vi "WLC Fitting For OneDirectionOnly_YCC.vi"() -> ()   [LabVIEW 2014]
uses:
  SubVI/WLC-Fitting Cluster.ctl
  <vilib>/Utility/file.llb/Read From Spreadsheet File (DBL).vi
  <vilib>/gmath/NumericalOptimization/Nonlinear Curve Fit LM formula string.vi
  <vilib>/Utility/file.llb/Write To Spreadsheet File (DBL).vi
  <vilib>/gmath/NI_Gmath.lvlib
panel:
  out "F-Force":dbl[](array[numeric])
  out "F-xDNA":dbl[](array[numeric])
  in  "F-yr shift (mV)":dbl
  in  "F-cr shift (nm)":dbl
  out "F-QPD signal (V)":dbl[](array[numeric])
  out "F-Stage Positions (um)":dbl[](array[numeric])
  in  "stuckbead path (dialog if empty)":path
  in  "F+U data?":bool
  in  "Ready to Fit":bool
  out "Save to Path":path
  out "best nonlinear fit force":dbl[](array[numeric])
  in  "SaveName":enum16{"ForecExtension Only", "WLC Fitting"}(ring)
  in  "Save Data?":bool
  in  "Finish Fitting":bool
  out "best fit parameters":dbl[](array[numeric])
  in  "initial parameters 2":dbl[](array[numeric])=[40.0, 1150.0]
  in  "Enum":T1(ring)
  in  "initial parameters for fit K":dbl[](array[numeric])=[40.0, 1150.0]
  out "U-Force":dbl[](array[numeric])
  out "U-xDNA":dbl[](array[numeric])
  out "Fitting Cluster for indicator":T2={"cr (um)"=0.0, "yr (V)"=0.0, "trap height(nm)"=0.0, "bead radius(nm)"=520.0, "Length offset"=0.0, "Force offset"=0.0, "cr shift (nm)"=0.0, "yr shift (mV)"=0.0, "LaserPower (mW)"=0.0, "conversion factor (V/um)"=0.0, "Stiffness (pN/nm)"=0.0154}
  in  "OneDirectionOnly?":bool=TRUE
  in  "Fitting Cluster for contorl":T2={"cr (um)"=0.0, "yr (V)"=0.0, "trap height(nm)"=200.0, "bead radius(nm)"=520.0, "Length offset"=0.0, "Force offset"=0.0, "cr shift (nm)"=0.0, "yr shift (mV)"=0.0, "LaserPower (mW)"=0.0, "conversion factor (V/um)"=0.0, "Stiffness (pN/nm)"=0.0154}
  in  "Tab Control":T3(tab)
  out "Stage-QPD Graph":T4(graph)
  out "U-Extension-Force Graph":cluster{"xDNA":dbl[], "Force":dbl[]}(graph)
  out "F-Extension-Force Graph":cluster{"xDNA":dbl[], "Force":dbl[]}(graph)
  out "All-Extension-Force Graph":T5(graph)
  out "Extension-Force and WLC Graph":cluster{"xDNA":dbl[], "Force":dbl[]}[](graph)
  out "Cut Stage Position (um)":dbl[](array[numeric])
  out "Cut QPD (V)":dbl[](array[numeric])
  in  "Delete Outside Signal?":bool
  out "U-QPD signal (V)":dbl[](array[numeric])
  out "U-Stage Positions (um)":dbl[](array[numeric])
  in  "Load Stage-QPD data":path
  in  "QPD":dbl[](array[numeric])
  in  "Stage":dbl[](array[numeric])
  in  "T=Read data mode?\nF=Real time fit":bool=TRUE
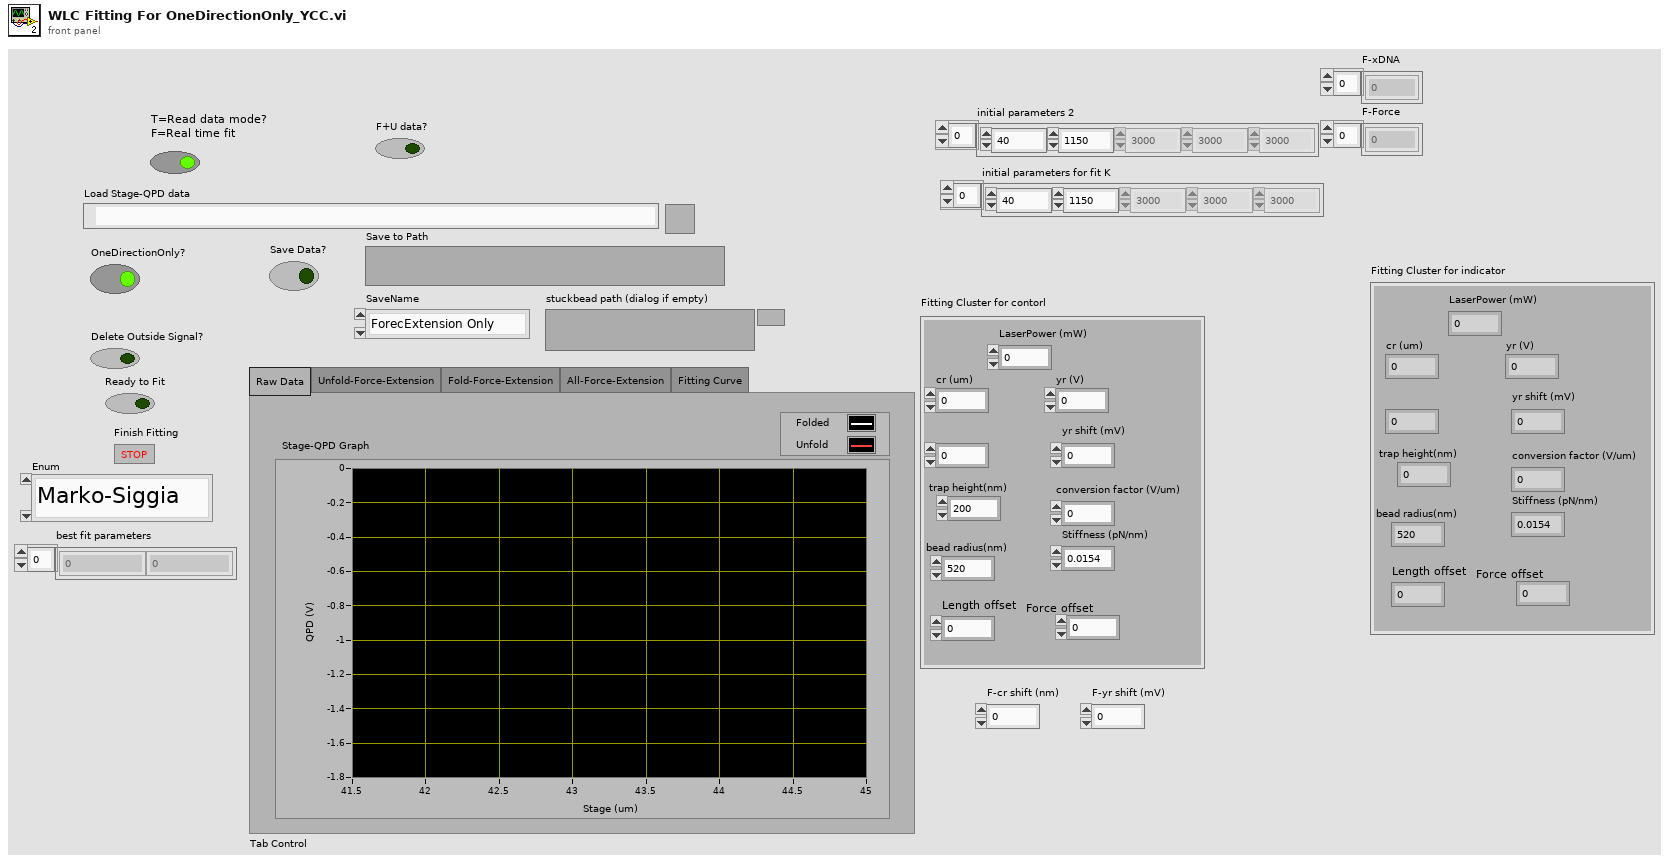
[diagram p1: front panel]
types:
  T1 = enum16{"Marko-Siggia", "modified Marko", "eWLC", "eWLC-modified M-S", "K fit eWLC-modified M-S"}
  T2 = typedef "WLC-Fitting Cluster.ctl" = cluster{"cr (um)":dbl, "yr (V)":dbl, "trap height(nm)":dbl, "bead radius(nm)":dbl, "Length offset":dbl, "Force offset":dbl, "cr shift (nm)":dbl, "yr shift (mV)":dbl, "LaserPower (mW)":dbl, "conversion factor (V/um)":dbl, "Stiffness (pN/nm)":dbl}
  T3 = enum32{"Raw Data", "Unfold-Force-Extension", "Fold-Force-Extension", "All-Force-Extension", "Fitting Curve"}
  T4 = cluster{"Sorted Stage Position (um)":dbl[], "Sorted QPD (V)":dbl[]}[]
  T5 = cluster{"Folded-xDNA":dbl[], "Folded-Force":dbl[]}[]
  T6 = cluster{"model":string, "Parameters":string[], "x":string}
  T7 = cluster{"F-Stage Positions (um) ":dbl[], "F-QPD signal (V) ":dbl[]}
  T8 = cluster{"U-Stage Positions (um)":dbl[], "U-QPD signal (V)":dbl[]}
  T9 = cluster{"U-Stage Positions (um)":dbl[], "U-QPD signal (V)":dbl[]}[]
  T10 = cluster{"Unfolded-xDNA":dbl[], "Unfolded-Force":dbl[]}
  T11 = cluster{"Folded-xDNA":dbl[], "Folded-Force":dbl[]}
  T12 = cluster{"Unfolded-xDNA":dbl[], "Unfolded-Force":dbl[]}[]
  T13 = cluster{"U-xDNA":dbl[], "best nonlinear fit":dbl[]}
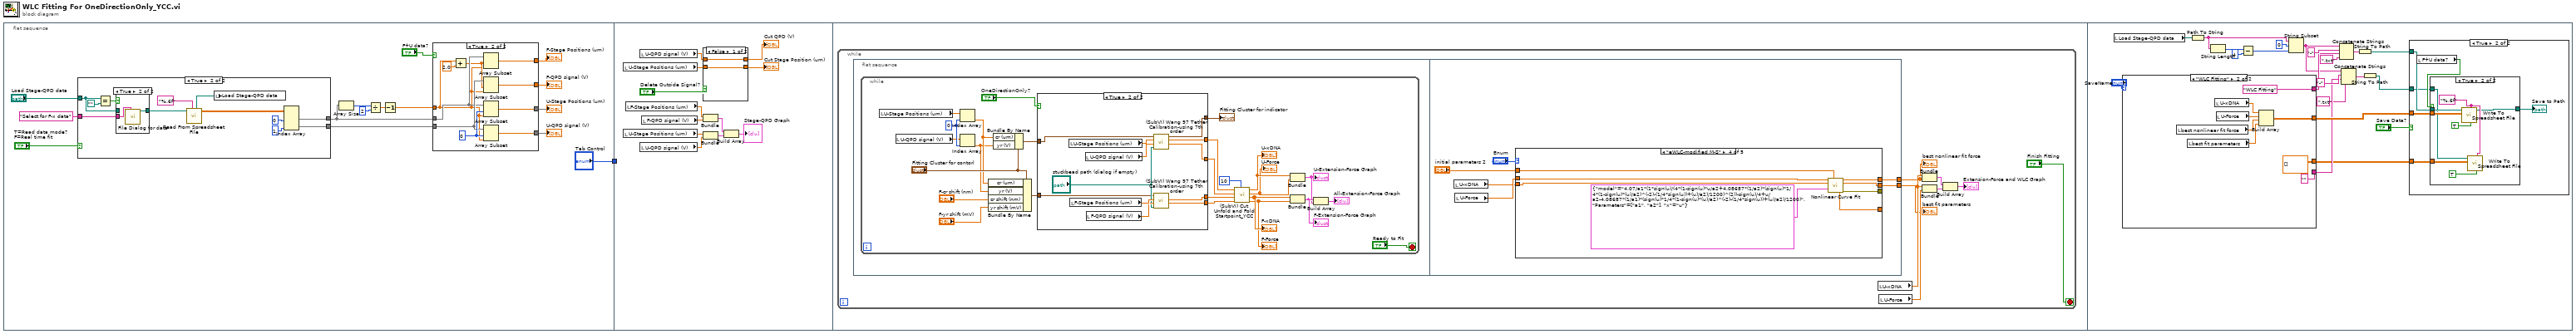
[diagram p0: block diagram]
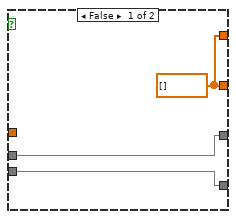
[diagram p2: hidden frame]
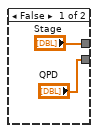
[diagram p3: hidden frame]
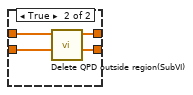
[diagram p5: hidden frame]
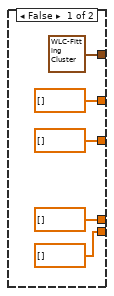
[diagram p6: hidden frame]
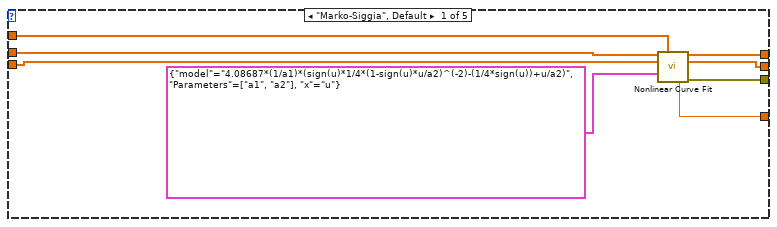
[diagram p7: hidden frame]
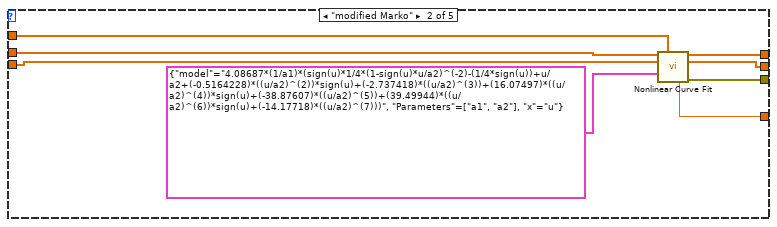
[diagram p8: hidden frame]
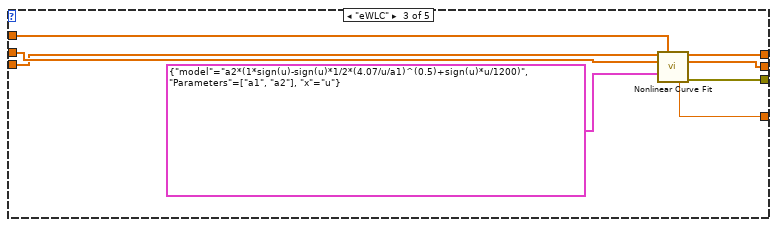
[diagram p9: hidden frame]
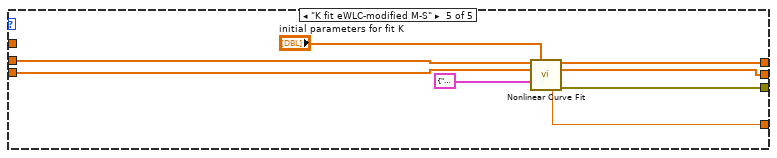
[diagram p10: hidden frame]
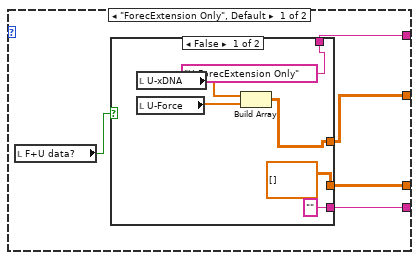
[diagram p11: hidden frame]
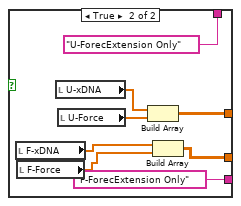
[diagram p12: hidden frame]
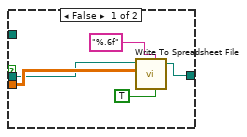
[diagram p14: hidden frame]
diagram:
  n1 = flat-sequence {
    tunnel: ["Tab Control"] -> w1
    tunnel: w1 -> [_]
    frame #0 {
      n2 = case shown="True" "T=Read data mode?\nF=Real time fit" {
        tunnel: ["QPD" w39] -> w11
        tunnel: ["Stage" w40] -> w6
        tunnel: "Select for F-x data" ("default name") -> [_ w36]
        tunnel: "Load Stage-QPD data" -> [_ w33]
        frame False {
        }
        frame True {
          n3 = Equal?(x=w33, y=path "") -> (x = y?=w34:bool)
          n4 = case shown="True" w34 {
            tunnel: [w44 w45] -> w37
            tunnel: w36 -> [_ w46]
            tunnel: w33 -> [w44 _]
            frame False {
            }
            frame True {
              n5 = call "File Dialog for data"("prompt"=w46) -> ("selected path"=w45:path)  [unwired: 11 in, 3 out]
            }
          }
          n6 = call-poly <vilib>:"Read From Spreadsheet File.vi"("format (%.3f)"="%.6f", "file path (dialog if empty)"=w37) -> ("all rows"=w43:dbl[][], "new file path (Not A Path if cancelled)"=w32:path)  [unwired: 5 in, 3 out]
          n7 = local write "Load Stage-QPD data"(w32) -> ()
          n8 = Index Array(array=w43, index (col) #1=0 ("disabled index (col)"), index (col) #2=1 ("index (col)")) -> (element #1=w40:dbl[], element #2=w39:dbl[])  [unwired: 2 in]
        }
      }
      n9 = Array Size(array=w6) -> (size(s)=w7:i32)
      n10 = Divide(x=w7, y=2) -> (x/y=w5:dbl)
      n11 = Decrement(x=w5) -> (x-1=w4:dbl)
      n12 = case shown="True" "F+U data?" {
        tunnel: w6 -> [w19 w25]
        tunnel: w11 -> [w18 w26]
        tunnel: [w19 w29] -> w10
        tunnel: [w18 w27] -> w9
        tunnel: w4 -> [_ w20]
        tunnel: [w17 w24] -> w3
        tunnel: [w17 w23] -> w2
        frame False {
          w17 = dbl[] []
        }
        frame True {
          w28 = 0 ("index")
          n13 = Add(x=w20, y=2.0) -> (x+y=w21:dbl)
          n14 = Array Subset(array=w25, index=w21, length=w20) -> (w24:dbl[])
          n15 = Array Subset(array=w26, index=w21, length=w20) -> (w23:dbl[])
          n16 = Array Subset(array=w25, index=w28, length=w20) -> (w29:dbl[])
          n17 = Array Subset(array=w26, index=w28, length=w20) -> (w27:dbl[])
        }
      }
      "U-Stage Positions (um)" <- w10
      "U-QPD signal (V)" <- w9
      "F-Stage Positions (um)" <- w3
      "F-QPD signal (V)" <- w2
    }
    frame #1 {
      n18 = local read "U-Stage Positions (um)"() -> (w57:dbl[])
      n19 = local read "U-Stage Positions (um)"() -> (w55:dbl[])
      n20 = local read "F-Stage Positions (um)"() -> (w48:dbl[])
      n21 = local read "U-QPD signal (V)"() -> (w56:dbl[])
      n22 = local read "U-QPD signal (V)"() -> (w54:dbl[])
      n23 = local read "F-QPD signal (V)"() -> (w47:dbl[])
      n24 = case shown="False" "Delete Outside Signal?" {
        tunnel: w56 -> [w60 w64]
        tunnel: w57 -> [w59 w63]
        tunnel: [w60 w62] -> w49
        tunnel: [w59 w61] -> w50
        frame False {
        }
        frame True {
          n25 = call "Delete QPD outside region(SubVI).vi"("Position Array In"=w63, "QPD signal In"=w64) -> ("Position Array Out"=w61:dbl[], "QPD signal Out"=w62:dbl[])  [unwired: 8 in]
        }
      }
      "Cut QPD (V)" <- w49
      "Cut Stage Position (um)" <- w50
      n26 = Bundle("F-Stage Positions (um)"=w48, "F-QPD signal (V)"=w47) -> (w53:T7)  [unwired: 1 in]
      n27 = Bundle("U-Stage Positions (um)"=w55, "U-QPD signal (V)"=w54) -> (w52:T8)  [unwired: 1 in]
      n28 = Build Array(w53, w52) -> (→"Stage-QPD Graph":T9)
    }
    frame #2 {
      n29 = while {
        stop <- "Finish Fitting" stop-if-true
        n30 = flat-sequence {
          tunnel: [w116] -> w66
          tunnel: [w115] -> w65
          frame #0 {
            n31 = while {
              stop <- "Ready to Fit" stop-if-true
              w96 = 0 ("index")
              n32 = local read "U-Stage Positions (um)"() -> (w87:dbl[])
              n33 = local read "U-QPD signal (V)"() -> (w86:dbl[])
              n34 = Index Array(array=w87, index=w96) -> (element=w84:dbl)
              n35 = Index Array(array=w86, index=w96) -> (element=w83:dbl)
              n36 = Bundle By Name(cluster="Fitting Cluster for contorl", "cr (um)"=w84, "yr (V)"=w83, "cr shift (nm)"="F-cr shift (nm)", "yr shift (mV)"="F-yr shift (mV)") -> (w80:T2)
              n37 = Bundle By Name(cluster="Fitting Cluster for contorl", "cr (um)"=w84, "yr (V)"=w83) -> (w95:T2)
              n38 = case shown="True" "OneDirectionOnly?" {
                tunnel: w95 -> [_ w110]
                tunnel: [T2 {"cr (um)"=0.0, "yr (V)"=0.0, "trap height(nm)"=0.0, "bead radius(nm)"=520.0, "Length offset"=0.0, "Force offset"=0.0, "cr shift (nm)"=0.0, "yr shift (mV)"=0.0, "LaserPower (mW)"=0.0, "conversion factor (V/um)"=0.0, "Stiffness (pN/nm)"=0.0154} ("Fitting Cluster for contorl") w111] -> w94
                tunnel: [dbl[] [] ("xDNA") w113] -> w91
                tunnel: [dbl[] [] ("Force") w112] -> w90
                tunnel: w80 -> [_ w105]
                tunnel: [dbl[] [] ("xDNA") w104] -> w79
                tunnel: [dbl[] [] ("xDNA") w103] -> w78
                frame False {
                }
                frame True {
                  n39 = local read "U-Stage Positions (um)"() -> (w109:dbl[])
                  n40 = local read "F-Stage Positions (um)"() -> (w108:dbl[])
                  n41 = local read "U-QPD signal (V)"() -> (w114:dbl[])
                  n42 = local read "F-QPD signal (V)"() -> (w107:dbl[])
                  n43 = call "(SubVI) Wang 97 Tether Calibration-using 7th order.vi"("stuckbead path (dialog if empty)"="stuckbead path (dialog if empty)", "QPD signal"=w114, "Stage Position"=w109, "Fitting Cluster"=w110) -> ("Force"=w112:dbl[], "xDNA"=w113:dbl[], "output cluster"=w111:T2)  [unwired: 3 in, 2 out]
                  n44 = call "(SubVI) Wang 97 Tether Calibration-using 7th order.vi"("stuckbead path (dialog if empty)"="stuckbead path (dialog if empty)", "QPD signal"=w107, "Stage Position"=w108, "Fitting Cluster"=w105) -> ("Force"=w103:dbl[], "xDNA"=w104:dbl[])  [unwired: 3 in, 3 out]
                }
              }
              "Fitting Cluster for indicator" <- w94
              n45 = call "(SubVI) Cut Unfold and Fold Startpoint_YCC.vi"("number to cut"=10, "Folded-Force in"=w78, "Folded-xDNA in"=w79, "Unfolded-Force"=w90, "Unfolded-xDNA"=w91) -> ("Folded-Force"=w73:dbl[], "Folded-xDNA"=w74:dbl[], "Unfolded-Force"=w88:dbl[], "Unfolded-xDNA"=w89:dbl[])  [unwired: 3 in]
              "U-xDNA" <- w89
              "U-Force" <- w88
              "F-xDNA" <- w74
              "F-Force" <- w73
              n46 = Bundle("Unfolded-xDNA"=w89, "Unfolded-Force"=w88) -> (w75:T10)  [unwired: 1 in]
              "U-Extension-Force Graph" <- w75
              n47 = Bundle("Folded-xDNA"=w74, "Folded-Force"=w73) -> (w76:T11)  [unwired: 1 in]
              "F-Extension-Force Graph" <- w76
              n48 = Build Array(w76, w75) -> (→"All-Extension-Force Graph":T12)
            }
          }
          frame #1 {
            n49 = local read "U-xDNA"() -> (w118:dbl[])
            n50 = local read "U-Force"() -> (w119:dbl[])
            n51 = case shown="\"eWLC-modified M-S\"" "Enum" {
              tunnel: "initial parameters 2" -> [w122 w135 w141 w151 _]
              tunnel: w119 -> [w127 w133 w143 w149 w159]
              tunnel: w118 -> [w121 w134 w142 w150 w158]
              tunnel: [w126 w130 w139 w145 w153] -> w116
              tunnel: [w125 w131 w140 w146 w154] -> w115
              tunnel: [w124 w132 w138 w147 w155] -> _
              tunnel: [w123 w129 w137 w148 w156] -> _
              frame "Marko-Siggia", Default {
                n52 = call-poly <vilib>:"Nonlinear Curve Fit.vi"("Y"=w127, "initial parameters"=w122, "X"=w121, "model description"=T6 {"model"="4.08687*(1/a1)*(sign(u)*1/4*(1-sign(u)*u/a2)^(-2)-(1/4*sign(u))+u/a2)", "Parameters"=["a1", "a2"], "x"="u"}) -> ("best nonlinear fit"=w126:dbl[], "best fit parameters"=w125:dbl[], "residue"=w123:dbl, "error out"=w124:errorcluster)  [unwired: 3 in, 5 out]
              }
              frame "modified Marko" {
                n53 = call-poly <vilib>:"Nonlinear Curve Fit.vi"("Y"=w133, "initial parameters"=w135, "X"=w134, "model description"=T6 {"model"="4.08687*(1/a1)*(sign(u)*1/4*(1-sign(u)*u/a2)^(-2)-(1/4*sign(u))+u/a2+(-0.5164228)*((u/a2)^(2))*sign(u)+(-2.737418)*((u/a2)^(3))+(16.07497)*((u/a2)^(4))*sign(u)+(-38.87607)*((u/a2)^(5))+(39.49944)*((u/a2)^(6))*sign(u)+(-14.17718)*((u/a2)^(7)))", "Parameters"=["a1", "a2"], "x"="u"}) -> ("best nonlinear fit"=w130:dbl[], "best fit parameters"=w131:dbl[], "residue"=w129:dbl, "error out"=w132:errorcluster)  [unwired: 3 in, 5 out]
              }
              frame "eWLC" {
                n54 = call-poly <vilib>:"Nonlinear Curve Fit.vi"("Y"=w142, "initial parameters"=w141, "X"=w143, "model description"=T6 {"model"="a2*(1*sign(u)-sign(u)*1/2*(4.07/u/a1)^(0.5)+sign(u)*u/1200)", "Parameters"=["a1", "a2"], "x"="u"}) -> ("best nonlinear fit"=w139:dbl[], "best fit parameters"=w140:dbl[], "residue"=w137:dbl, "error out"=w138:errorcluster)  [unwired: 3 in, 5 out]
              }
              frame "eWLC-modified M-S" {
                n55 = call-poly <vilib>:"Nonlinear Curve Fit.vi"("Y"=w149, "initial parameters"=w151, "X"=w150, "model description"=T6 {"model"="4.07/a1*(1*sign(u)/(4*(1-sign(u)*u/a2+4.08687*(1/a2)*(sign(u)*1/4*(1-sign(u)*(u)/a2)^(-2)-(1/4*sign(u))+(u)/a2)/1200)^(2))-sign(u)/4+u/a2-4.08687*(1/a1)*(sign(u)*1/4*(1-sign(u)*(u)/a2)^(-2)-(1/4*sign(u))+(u)/a2)/1200)", "Parameters"=["a1", "a2"], "x"="u"}) -> ("best nonlinear fit"=w145:dbl[], "best fit parameters"=w146:dbl[], "residue"=w148:dbl, "error out"=w147:errorcluster)  [unwired: 7 in, 1 out]
              }
              frame "K fit eWLC-modified M-S" {
                n56 = call-poly <vilib>:"Nonlinear Curve Fit.vi"("Y"=w159, "initial parameters"="initial parameters for fit K", "X"=w158, "model description"=T6 {"model"="4.07/a1*(1*sign(u)/(4*(1-sign(u)*u/a2+4.08687*(1/a2)*(sign(u)*1/4*(1-sign(u)*(u)/a2)^(-2)-(1/4*sign(u))+(u)/a2)/a3)^(2))-sign(u)/4+u/a2-4.08687*(1/a1)*(sign(u)*1/4*(1-sign(u)*(u)/a2)^(-2)-(1/4*sign(u))+(u)/a2)/a3)", "Parameters"=["a1", "a2", "a3"], "x"="u"}) -> ("best nonlinear fit"=w153:dbl[], "best fit parameters"=w154:dbl[], "residue"=w156:dbl, "error out"=w155:errorcluster)  [unwired: 7 in, 1 out]
              }
            }
          }
        }
        n57 = local read "U-xDNA"() -> (w71:dbl[])
        n58 = local read "U-Force"() -> (w70:dbl[])
        n59 = Bundle("U-xDNA"=w71, "best nonlinear fit"=w66) -> (w69:T13)  [unwired: 1 in]
        n60 = Bundle("U-xDNA"=w71, "U-Force"=w70) -> (w68:cluster{"U-xDNA":dbl[], "U-Force":dbl[]})  [unwired: 1 in]
        n61 = Build Array(w69, w68) -> (→"Extension-Force and WLC Graph":cluster{"U-xDNA":dbl[], "U-Force":dbl[]}[])
        "best nonlinear fit force" <- w66
        "best fit parameters" <- w65
      }
    }
    frame #3 {
      n62 = local read "Load Stage-QPD data"() -> (w181:path)
      n63 = case shown="\"WLC Fitting\"" "SaveName" {
        tunnel: [w186 "WLC Fitting" ("string")] -> w172
        tunnel: [w185 w203] -> w169
        tunnel: [w183 "" ("string")] -> w164
        tunnel: [w182 dbl[][] []] -> w161
        frame "ForecExtension Only", Default {
          n64 = local read "F+U data?"() -> (w184:bool)
          n65 = case shown="False" w184 {
            tunnel: ["U-ForecExtension Only" ("string") "U-ForecExtension Only" ("string")] -> w186
            tunnel: [w187 w197] -> w185
            tunnel: ["" ("string") "F-ForecExtension Only" ("string")] -> w183
            tunnel: [dbl[][] [] w193] -> w182
            frame False {
              n66 = local read "U-xDNA"() -> (w189:dbl[])
              n67 = local read "U-Force"() -> (w188:dbl[])
              n68 = Build Array(w189, w188) -> (w187:dbl[][])
            }
            frame True {
              n69 = local read "F-xDNA"() -> (w196:dbl[])
              n70 = local read "F-Force"() -> (w195:dbl[])
              n71 = local read "U-xDNA"() -> (w199:dbl[])
              n72 = local read "U-Force"() -> (w198:dbl[])
              n73 = Build Array(w199, w198) -> (w197:dbl[][])
              n74 = Build Array(w196, w195) -> (w193:dbl[][])
            }
          }
        }
        frame "WLC Fitting" {
          n75 = local read "best nonlinear fit force"() -> (w205:dbl[])
          n76 = local read "best fit parameters"() -> (w204:dbl[])
          n77 = local read "U-xDNA"() -> (w207:dbl[])
          n78 = local read "U-Force"() -> (w206:dbl[])
          n79 = Build Array(w207, w206, w205, w204) -> (w203:dbl[][])
        }
      }
      n80 = Path To String(path=w181) -> (string=w179:string)
      n81 = String Length(string=w179) -> (length=w178:i32)
      n82 = Subtract(x=w178, y=4) -> (x-y=w175:i32)
      n83 = String Subset(string=w179, offset (0)=0, length (rest)=w175) -> (substring=w166:string)
      n84 = Concatenate Strings(w166, "-" ("string"), w172, ".txt" ("string")) -> (w168:string)
      n85 = Concatenate Strings(w166, "-" ("string"), w164, ".txt" ("string")) -> (w167:string)
      n86 = String To Path(string=w168) -> (path=w170:path)
      n87 = String To Path(string=w167) -> (path=w162:path)
      n88 = case shown="True" "Save Data?" {
        tunnel: w170 -> [_ w214]
        tunnel: w169 -> [_ w213]
        tunnel: w162 -> [_ w211]
        tunnel: w161 -> [_ w210]
        frame False {
        }
        frame True {
          n89 = local read "F+U data?"() -> (w212:bool)
          n90 = case shown="True" w212 {
            tunnel: w214 -> [w216 w227]
            tunnel: w213 -> [w217 w226]
            tunnel: w211 -> [_ w223]
            tunnel: w210 -> [_ w222]
            tunnel: [w215 w220] -> w209
            frame False {
              n91 = call-poly <vilib>:"Write To Spreadsheet File.vi"("transpose? (no:F)"=TRUE, "format (%.3f)"="%.6f", "2D data"=w217, "file path (dialog if empty)"=w216) -> ("new file path (Not A Path if cancelled)"=w215:path)  [unwired: 4 in]
            }
            frame True {
              w224 = "%.6f" ("format (%.3f)")
              n92 = call-poly <vilib>:"Write To Spreadsheet File.vi"("transpose? (no:F)"=TRUE, "format (%.3f)"=w224, "2D data"=w226, "file path (dialog if empty)"=w227) -> ("new file path (Not A Path if cancelled)"=w220:path)  [unwired: 4 in]
              n93 = call-poly <vilib>:"Write To Spreadsheet File.vi"("transpose? (no:F)"=TRUE, "format (%.3f)"=w224, "2D data"=w222, "file path (dialog if empty)"=w223) -> ()  [unwired: 4 in, 1 out]
            }
          }
          "Save to Path" <- w209
        }
      }
    }
  }
